vi "Slow Move.vi"(8 "error in (no error)":errorcluster, 11 "ScrollingList in":refnum<class "ScrollingList.lvclass">) -> (0 "error out":errorcluster, 3 "ScrollingList out":refnum<class "ScrollingList.lvclass">)   [LabVIEW 2020, in "ScrollingList.lvclass"]
uses:
  ScrollingList.lvclass
  ScrollingList.lvclass/ScrollingList.ctl
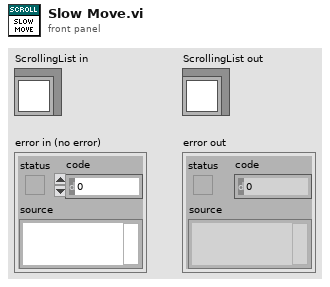
[diagram p1: front panel]
types:
  T1 = typedef "ScrollingList.lvclass/State Data.ctl" = cluster{"Timeout":i32, "Time":timestamp, "Y":i32, "Origin:Top":i16, "Rate":dbl, "ListItems":string[], "Item Height":i32, "Max Height":i32}
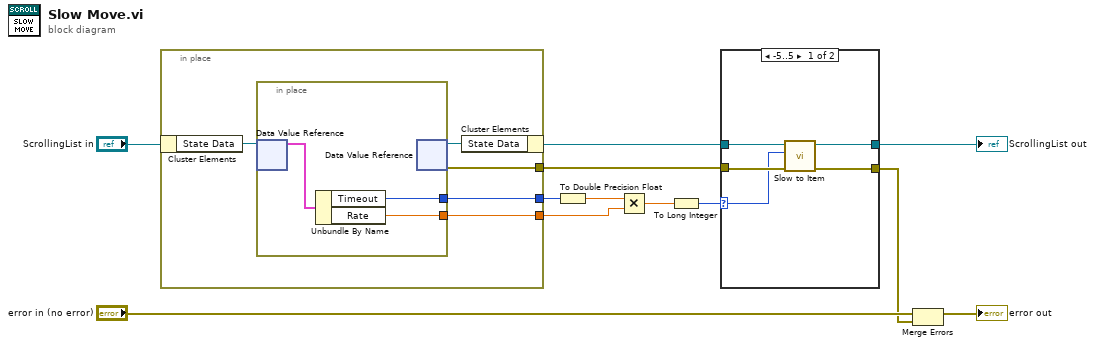
[diagram p0: block diagram]
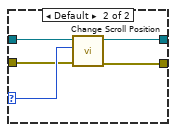
[diagram p2: hidden frame]
diagram:
  n1 = in-place {
    in-place-border: [w16] -> w8
    in-place-border: [w14] -> w7
    in-place-border: [w13] -> w4
    n2 = in-place-cluster #1("ScrollingList in") -> ("State Data"=w17:refnum<data-value>)
    n3 = in-place {
      in-place-border: [w19] -> w16
      in-place-border: [w18] -> w14
      n4 = in-place-dvr #2(w17) -> (w20:T1)  [unwired: 1 out]
      n5 = Unbundle By Name(w20) -> ("Timeout"=w19:i32, "Rate"=w18:dbl)
      n6 = in-place-dvr #2() -> (w15:refnum<data-value>, w13:errorcluster)  [unwired: 1 in]
    }
    n7 = in-place-cluster #1("State Data"=w15) -> (w5:refnum<class "ScrollingList.lvclass">)
  }
  n8 = To Double Precision Float(number=w8) -> (double precision float=w9:dbl)
  n9 = Multiply(x=w9, y=w7) -> (x*y=w10:dbl)
  n10 = To Long Integer(number=w10) -> (32bit integer=w6:i32)
  n11 = case shown="-5..5" w6 {
    selector: w6 -> [w22 w29]
    tunnel: w5 -> [w25 w30]
    tunnel: w4 -> [w23 w28]
    tunnel: [w24 w27] -> w3
    tunnel: [w21 w26] -> w1
    frame -5..5 {
      n12 = call "Slow to Item.vi"("error in (no error)"=w23, "Position Change"=w22, "ScrollingList in"=w25) -> ("error out"=w21:errorcluster, "ScrollingList out"=w24:refnum<class "ScrollingList.lvclass">)  [unwired: 7 in]
    }
    frame Default {
      n13 = call "Change Scroll Position.vi"("error in (no error)"=w28, "Position Change"=w29, "ScrollingList in"=w30) -> ("error out"=w26:errorcluster, "ScrollingList out"=w27:refnum<class "ScrollingList.lvclass">)  [unwired: 7 in]
    }
  }
  "ScrollingList out" <- w3
  n14 = Merge Errors("error in (no error)", w1) -> (→"error out":errorcluster)
